vi "Test_IncrementValuePublication_DBL_ValueIncremented.vi"(8 "error in (no error)":errorcluster, 11 "TestCase in":refnum<class "TestPublicationPolicy.lvclass">) -> (0 "error out":errorcluster, 3 "TestCase out":refnum<class "TestPublicationPolicy.lvclass">)   [LabVIEW 2015, in "PublicationPolicy.lvlib" / "TestPublicationPolicy.lvclass"]
uses:
  TestPublicationPolicy.lvclass
  IncrementValuePublication/IncrementValuePublication.lvclass
  IMediator/IPublicationPolicy/IPublicationPolicy.lvclass
  Transport/QueueTransport/QueueTransport.lvclass/QueueTransport.ctl
  IMediator/PublishRequest/PublishRequest.lvclass/PublishRequest.ctl
  IMediator/MutexedPublishRequest/MutexedPublishRequest.lvclass/MutexedPublishRequest.ctl
  IMediator/PublishRequest/Write Publish Request Data.vi
  <vilib>/Utility/error.llb/Error Cluster From Error Code.vi
  IMediator/MutexedPublishRequest/MutexedPublishRequest.lvclass
  Transport/QueueTransport/QueueTransport.lvclass
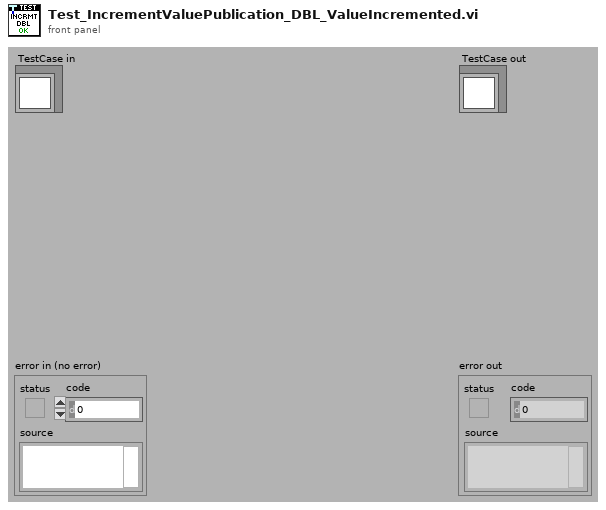
[diagram p1: front panel]
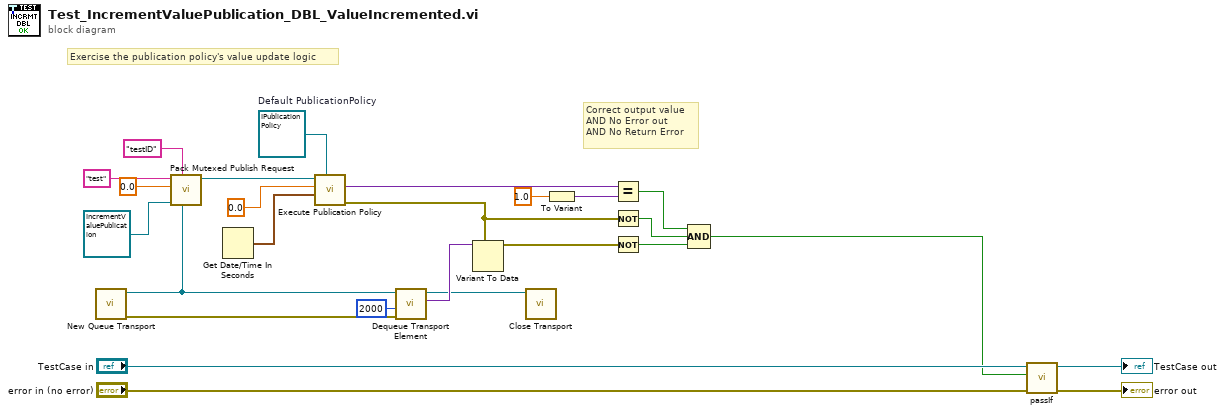
[diagram p0: block diagram]
diagram:
  w18 = refnum<class "IPublicationPolicy.lvclass"> refnum  # Default PublicationPolicy
  # "Correct output value\nAND No Error out\nAND No Return Error"
  # "Exercise the publication policy's value update logic"
  n1 = call "New Queue Transport.vi"() -> ("error out"=w13:errorcluster, "QueueTransport"=w14:refnum<class "QueueTransport.lvclass">)  [unwired: 10 in]
  n2 = call "Pack Mutexed Publish Request.vi"("Return Error Transport"=w14, "Publisher ID"="testID", "PublicationPolicy"=refnum<class "IncrementValuePublication.lvclass"> refnum ("PublicationPolicy.lvlib:IncrementValuePublication.lvclass"), "Datum Value or Type"=0.0 ("Data to Publish"), "Datum Name"="test") -> ("MutexedPublishRequest Out"=w20:refnum<class "MutexedPublishRequest.lvclass">)  [unwired: 6 in]
  n3 = Get Date/Time In Seconds() -> (seconds since 1Jan1904=w21:timestamp)
  n4 = call-dynamic "Execute Publication Policy.vi"("Default PublicationPolicy"=w18, "Last Publish Time"=w21, "Last Published Value"=0.0, "MutexedPublishRequest"=w20) -> ("error out (Reject Publication)"=w2:errorcluster, "Value to Publish"=w10:variant)  [unwired: 5 in, 1 out]
  n5 = call "Dequeue Transport Element.vi"("error in (no error)"=w13, "Timeout In ms (-1)"=2000, "QueueTransport in"=w14) -> ("Data"=w11:variant, "QueueTransport out"=w6:refnum<class "QueueTransport.lvclass">)  [unwired: 5 in, 2 out]
  n6 = Variant To Data(type=w2, Variant=w11) -> (data=w7:errorcluster)  [unwired: 1 in, 1 out]
  n7 = call-dynamic "Close Transport.vi"("QueueTransport in"=w6) -> ()  [unwired: 10 in, 1 out]
  n8 = To Variant(anything=1.0) -> (Variant=w8:variant)
  n9 = Equal?(x=w10, y=w8) -> (x = y?=w5:bool)
  n10 = Not(x=w2) -> (.not. x?=w1:bool)
  n11 = Not(x=w7) -> (.not. x?=w3:bool)
  n12 = Compound Arithmetic op=AND(w5, w1, w3) -> (w4:bool)
  n13 = call-dynamic "passIf.vi"("error in (no error)"="error in (no error)", "pass"=w4, "TestCase in"="TestCase in") -> ("error out"=→"error out":errorcluster, "TestCase out"=→"TestCase out":refnum<class "TestPublicationPolicy.lvclass">)  [unwired: 7 in]
